vi "Is Open.vi"(8 "error in (no error)":errorcluster, 11 "Websocket Client in":refnum<class "Websocket Client.lvclass">) -> (0 "error out":errorcluster, 2 "Is Open":bool, 3 "Websocket Client out":refnum<class "Websocket Client.lvclass">)   [LabVIEW 2020, in "Stream-Websocket.lvlib" / "Websocket Client.lvclass"]
uses:
  Websocket Client.lvclass
  Websocket Client.lvclass/Websocket Client.ctl
  <vilib>/IlluminatedG/lv-stream/Connection/Connection.lvclass
  <vilib>/IlluminatedG/lv-stream/Connection/State.ctl
  C:/Program Files (x86)/National Instruments/LabVIEW 2020/vi.lib/IlluminatedG/lv-stream/Connection/Connection.lvclass
  C:/Program Files (x86)/National Instruments/LabVIEW 2020/vi.lib/IlluminatedG/lv-stream/Endpoint/Endpoint.lvclass
  C:/dev/illuminated-g/lv-stream-websocket/Stream-Websocket/Websocket Client/Websocket Client.lvclass
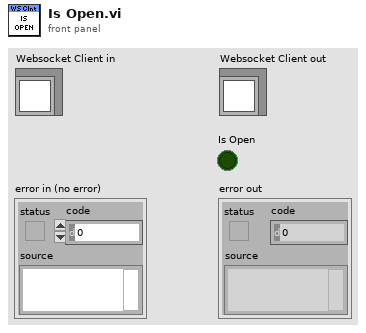
[diagram p1: front panel]
types:
  T1 = typedef "Stream.lvlib/Connection.lvclass/State.ctl" = enum16{"Closed", "Idle", "Connecting", "Connected", "Shutdown"}
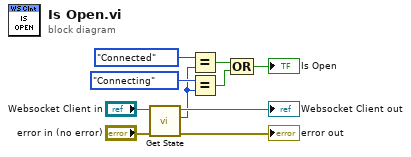
[diagram p0: block diagram]
diagram:
  n1 = call <vilib>:"Get State.vi"("error in (no error)"="error in (no error)", "Connection in"="Websocket Client in") -> ("error out"=→"error out":errorcluster, "State"=w5:T1, "Connection out"=→"Websocket Client out":refnum<class "Websocket Client.lvclass">)  [unwired: 7 in]
  n2 = Equal?(x=State."Connected", y=w5) -> (x = y?=w4:bool)
  n3 = Equal?(x=State."Connecting", y=w5) -> (x = y?=w3:bool)
  n4 = Compound Arithmetic op=OR(w4, w3) -> (→"Is Open":bool)
